vi "Initialize.vi"(7 "timeout, ms (300)":u32=300, 8 "error in (no error)":errorcluster, 10 "baud rate (57600)":u32=57600, 11 "port":refnum<visa-resource-name>) -> (0 "error out":errorcluster, 3 "Lotis out":refnum<class "PL Lotis TII LS.lvclass">)   [LabVIEW 2015, in "PL Lotis TII LS.lvclass"]
doc: "Initializes connection to device using specified settings."
uses:
  PL Lotis TII LS.lvclass
  PL Lotis TII LS.lvclass/PL Lotis TII LS.ctl
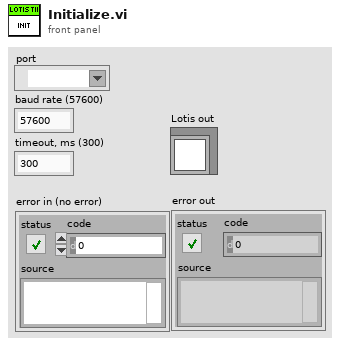
[diagram p1: front panel]
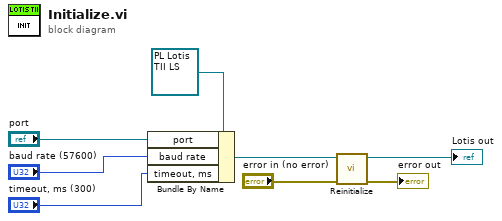
[diagram p0: block diagram]
diagram:
  n1 = Bundle By Name(cluster=refnum<class "PL Lotis TII LS.lvclass"> refnum ("PL Comdel CX.lvclass"), "port"="port", "baud rate"="baud rate (57600)", "timeout, ms"="timeout, ms (300)") -> (w8:refnum<class "PL Lotis TII LS.lvclass">)
  n2 = call "Reinitialize.vi"("error in (no error)"="error in (no error)", "Lotis in"=w8) -> ("error out"=→"error out":errorcluster, "Lotis out"=→"Lotis out":refnum<class "PL Lotis TII LS.lvclass">)  [unwired: 8 in]
